vi "Launcher.vi"   [LabVIEW 2019]
uses:
  Modules/Main/Main.lvlib
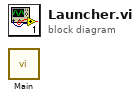
[diagram p0: block diagram]
diagram:
  n1 = call "Main.vi"() -> ()  [unwired: 12 in]
